vi "input user data.vi"() -> ()   [LabVIEW 2018]
panel:
  out "Output 7":string
  in  "Sample Serial #":string
  out "Output 6":string
  in  "Waveform Generator":string
  out "Output 5":string
  in  "Oscilloscope":string
  out "Output 4":string
  in  "Multimeter":string
  out "Output 3":string
  in  "Com Port":string
  out "Output 2":string
  in  "Station":string
  out "Output 1":string
  in  "User Name":string
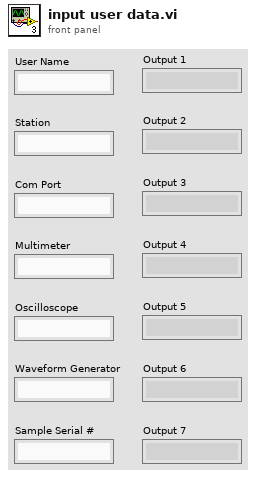
[diagram p1: front panel]
types:
  T1 = enum16{"Name", "Station", "Uart Com", "Multimeter", "Oscilliscope", "Waveform Generator", "Spec Sheet", "end"}
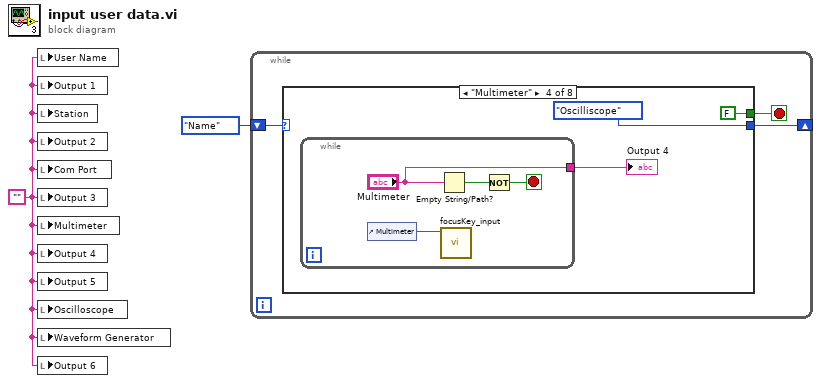
[diagram p0: block diagram]
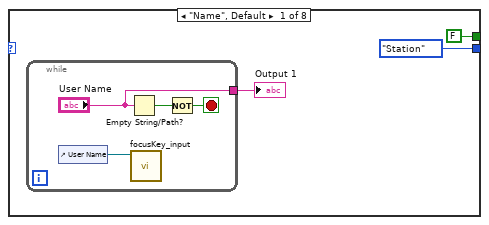
[diagram p2: hidden frame]
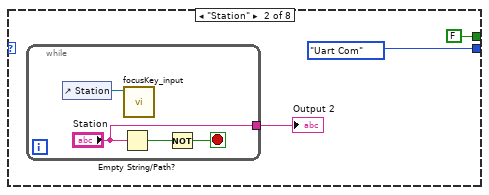
[diagram p3: hidden frame]
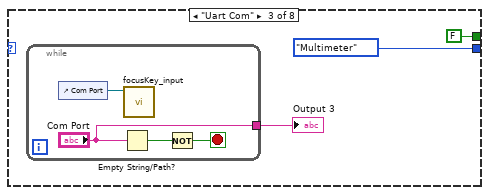
[diagram p4: hidden frame]
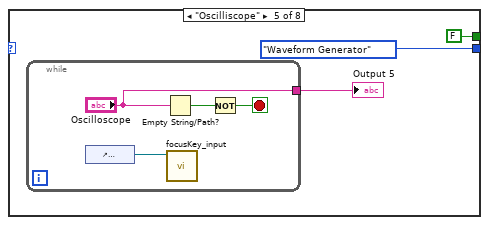
[diagram p5: hidden frame]
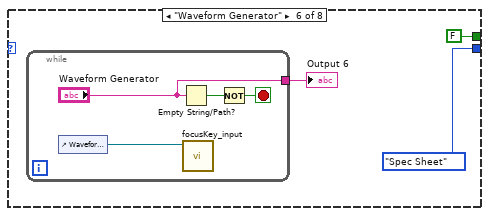
[diagram p6: hidden frame]
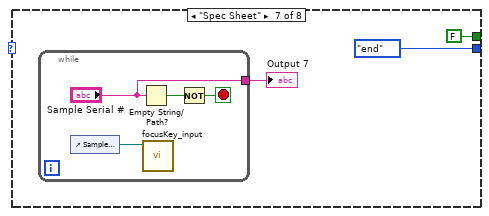
[diagram p7: hidden frame]
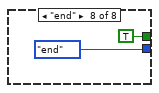
[diagram p8: hidden frame]
diagram:
  w1 = ""
  n1 = local write "User Name"(w1) -> ()
  n2 = local write "Output 1"(w1) -> ()
  n3 = local write "Station"(w1) -> ()
  n4 = local write "Output 2"(w1) -> ()
  n5 = local write "Com Port"(w1) -> ()
  n6 = local write "Output 3"(w1) -> ()
  n7 = local write "Multimeter"(w1) -> ()
  n8 = local write "Output 4"(w1) -> ()
  n9 = local write "Output 5"(w1) -> ()
  n10 = local write "Oscilloscope"(w1) -> ()
  n11 = local write "Waveform Generator"(w1) -> ()
  n12 = local write "Output 6"(w1) -> ()
  n13 = while {
    shift-right: [w4] -> _
    shift-left: T1."Name" -> [w5]
    stop <- w3 stop-if-true
    n14 = case shown="\"Multimeter\"" w5 {
      tunnel: [T1."Station" T1."Uart Com" T1."Multimeter" T1."Oscilliscope" T1."Waveform Generator" T1."Spec Sheet" T1."end" T1."end"] -> w4
      tunnel: [FALSE FALSE FALSE FALSE FALSE FALSE FALSE TRUE] -> w3
      frame "Name", Default {
        n15 = while {
          tunnel: ["User Name"] -> w8
          stop <- w11 stop-if-true
          n16 = control-ref of="User Name"() -> (w9:refnum<vi>)
          n17 = Empty String/Path?(string/path="User Name") -> (empty?=w12:bool)
          n18 = call "focusKey_input.vi"("reference"=w9) -> ()  [unwired: 10 in, 1 out]
          n19 = Not(x=w12) -> (.not. x?=w11:bool)
        }
        "Output 1" <- w8
      }
      frame "Station" {
        n20 = while {
          tunnel: ["Station"] -> w15
          stop <- w18 stop-if-true
          n21 = control-ref of="Station"() -> (w16:refnum<vi>)
          n22 = Empty String/Path?(string/path="Station") -> (empty?=w19:bool)
          n23 = call "focusKey_input.vi"("reference"=w16) -> ()  [unwired: 10 in, 1 out]
          n24 = Not(x=w19) -> (.not. x?=w18:bool)
        }
        "Output 2" <- w15
      }
      frame "Uart Com" {
        n25 = while {
          tunnel: ["Com Port"] -> w22
          stop <- w25 stop-if-true
          n26 = control-ref of="Com Port"() -> (w23:refnum<vi>)
          n27 = Empty String/Path?(string/path="Com Port") -> (empty?=w26:bool)
          n28 = call "focusKey_input.vi"("reference"=w23) -> ()  [unwired: 10 in, 1 out]
          n29 = Not(x=w26) -> (.not. x?=w25:bool)
        }
        "Output 3" <- w22
      }
      frame "Multimeter" {
        n30 = while {
          tunnel: ["Multimeter"] -> w29
          stop <- w32 stop-if-true
          n31 = control-ref of="Multimeter"() -> (w30:refnum<vi>)
          n32 = Empty String/Path?(string/path="Multimeter") -> (empty?=w33:bool)
          n33 = call "focusKey_input.vi"("reference"=w30) -> ()  [unwired: 10 in, 1 out]
          n34 = Not(x=w33) -> (.not. x?=w32:bool)
        }
        "Output 4" <- w29
      }
      frame "Oscilliscope" {
        n35 = while {
          tunnel: ["Oscilloscope"] -> w36
          stop <- w39 stop-if-true
          n36 = control-ref of="Oscilloscope"() -> (w37:refnum<vi>)
          n37 = Empty String/Path?(string/path="Oscilloscope") -> (empty?=w40:bool)
          n38 = call "focusKey_input.vi"("reference"=w37) -> ()  [unwired: 10 in, 1 out]
          n39 = Not(x=w40) -> (.not. x?=w39:bool)
        }
        "Output 5" <- w36
      }
      frame "Waveform Generator" {
        n40 = while {
          tunnel: ["Waveform Generator"] -> w43
          stop <- w46 stop-if-true
          n41 = control-ref of="Waveform Generator"() -> (w44:refnum<vi>)
          n42 = Empty String/Path?(string/path="Waveform Generator") -> (empty?=w47:bool)
          n43 = call "focusKey_input.vi"("reference"=w44) -> ()  [unwired: 10 in, 1 out]
          n44 = Not(x=w47) -> (.not. x?=w46:bool)
        }
        "Output 6" <- w43
      }
      frame "Spec Sheet" {
        n45 = while {
          tunnel: ["Sample Serial #"] -> w49
          stop <- w53 stop-if-true
          n46 = control-ref of="Sample Serial #"() -> (w51:refnum<vi>)
          n47 = Empty String/Path?(string/path="Sample Serial #") -> (empty?=w54:bool)
          n48 = call "focusKey_input.vi"("reference"=w51) -> ()  [unwired: 10 in, 1 out]
          n49 = Not(x=w54) -> (.not. x?=w53:bool)
        }
        "Output 7" <- w49
      }
      frame "end" {
      }
    }
  }
